vi "Node ID.vi"() -> ()   [LabVIEW 2016]
uses:
  Set Save Object Dictionary.vi
  Motor controllers.vi
  <vilib>/CANopenLib/CANOPEN.llb/CANopen SDO Create.vi
  Set node ID.vi
  Set PDOs COB IDs.vi
  Set COB EMCY ID.vi
  <vilib>/CANopenLib/CANOPEN.llb/CANopen SDO Write.vi
  <vilib>/CANopenLib/CANOPEN.llb/CANopen SDO Write [STR].vi
  <vilib>/CANopenLib/CANOPEN.llb/CANopen SDO Close.vi
  <vilib>/CANopenLib/CANOPEN.llb/CANopen Interface Close.vi
panel:
  in  "Motor":u8(ring) items=["Right", "Left"]
  in  "New Node ID":u8=1 min=1 max=127 step=1
  out "error out":errorcluster
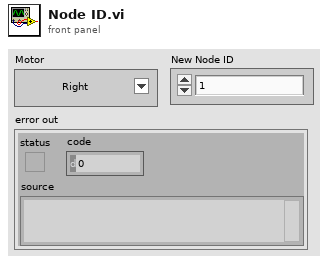
[diagram p1: front panel]
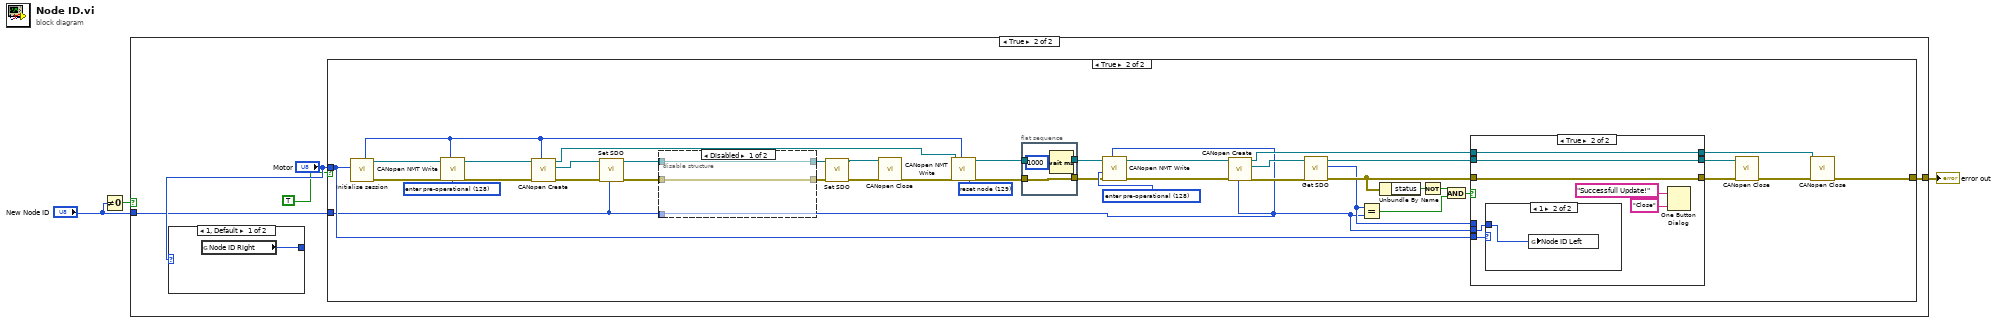
[diagram p0: block diagram]
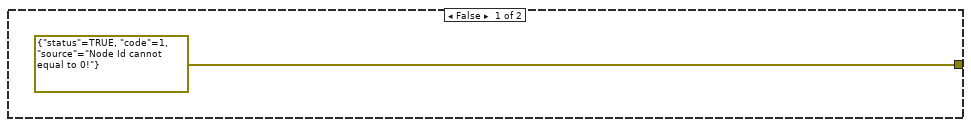
[diagram p2: hidden frame]
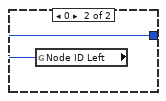
[diagram p3: hidden frame]
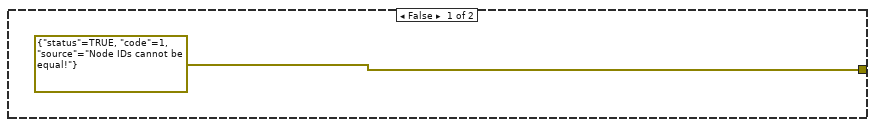
[diagram p4: hidden frame]
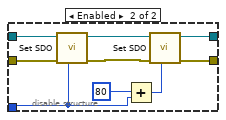
[diagram p5: hidden frame]
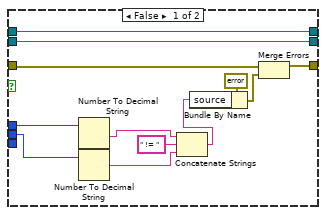
[diagram p6: hidden frame]
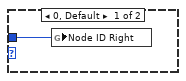
[diagram p7: hidden frame]
diagram:
  n1 = Not Equal To 0?(x="New Node ID") -> (x != 0?=w2:bool)
  n2 = case shown="True" w2 {
    tunnel: [errorcluster {"status"=TRUE, "code"=1, "source"="Node Id cannot equal to 0!"} ("error constant") w8] -> w3
    tunnel: "New Node ID" -> [_ w6]
    frame False {
    }
    frame True {
      n3 = case shown="1, Default" "Motor" {
        tunnel: [w9 w10] -> _
        frame 1, Default {
          n4 = global read "Motor controllers.vi" "Node ID Right"() -> (w9:u8)
        }
        frame 0 {
          n5 = global read "Motor controllers.vi" "Node ID Left"() -> (w10:u8)
        }
      }
      n6 = case shown="True" TRUE {
        tunnel: "Motor" -> [_ w49]
        tunnel: w6 -> [_ w16]
        tunnel: [errorcluster {"status"=TRUE, "code"=1, "source"="Node IDs cannot be equal!"} ("error constant") w35] -> w8
        frame False {
        }
        frame True {
          w21 = u16 128 items=["start remote node"=1, "stop remote node"=2, "enter pre-operational"=128, "reset node"=129, "reset communication"=130] ("command")
          w22 = u16 129 items=["start remote node"=1, "stop remote node"=2, "enter pre-operational"=128, "reset node"=129, "reset communication"=130] ("command")
          w50 = u16 128 items=["start remote node"=1, "stop remote node"=2, "enter pre-operational"=128, "reset node"=129, "reset communication"=130] ("command")
          n7 = call "Initialise session.vi"("Motor"=w49) -> ("error out"=w44:errorcluster, "interface object out"=w43:refnum<k20>, "Used Node ID"=w26:u8)  [unwired: 8 in]
          n8 = call <vilib>:"CANopen NMT Write.vi"("node-ID (0)"=w26, "error in (no error)"=w44, "command"=w50, "interface object in"=w43) -> ("error out"=w46:errorcluster, "interface object out"=w45:refnum<k20>)  [unwired: 6 in]
          n9 = call-poly <vilib>:"CANopen Create.vi"("node-ID"=w26, "error in (no error)"=w46, "interface object in"=w45) -> ("error out"=w52:errorcluster, "SDO object out"=w51:refnum<k20>, "interface object out"=w23:refnum<k20>)  [unwired: 6 in]
          n10 = call-poly "Set SDO.vi"("Node ID"=w16, "error in (no error)"=w52, "SDO object in"=w51) -> ("error out"=w20:errorcluster, "SDO object out"=w19:refnum<k20>)  [unwired: 6 in, 1 out]
          n11 = disable-structure shown="Disabled" {
            disable-tunnel: w20 -> [w53 w63]
            disable-tunnel: w19 -> [w54 w62]
            disable-tunnel: [w53 w59] -> w18
            disable-tunnel: [w54 w58] -> w17
            disable-tunnel: w16 -> [_ w56]
            frame Disabled {
            }
            frame Enabled {
              n12 = call-poly "Set SDO.vi"("Node ID"=w56, "error in (no error)"=w63, "SDO object in"=w62) -> ("error out"=w60:errorcluster, "SDO object out"=w61:refnum<k20>)  [unwired: 7 in]
              n13 = Add(x=u32 80, y=w56) -> (x+y=w55:u32)
              n14 = call-poly "Set SDO.vi"("COB EMCY ID"=w55, "error in (no error)"=w60, "SDO object in"=w61) -> ("error out"=w59:errorcluster, "SDO object out"=w58:refnum<k20>)  [unwired: 6 in, 1 out]
            }
          }
          n15 = call-poly "Set SDO.vi"("error in (no error)"=w18, "SDO object in"=w17) -> ("error out"=w28:errorcluster, "SDO object out"=w29:refnum<k20>)  [unwired: 7 in, 1 out]
          n16 = call-poly <vilib>:"CANopen Close.vi"("error in (no error)"=w28, "SDO object in"=w29) -> ("error out"=w27:errorcluster)  [unwired: 9 in]
          n17 = call <vilib>:"CANopen NMT Write.vi"("node-ID (0)"=w26, "error in (no error)"=w27, "command"=w22, "interface object in"=w23) -> ("error out"=w12:errorcluster, "interface object out"=w14:refnum<k20>)  [unwired: 6 in]
          n18 = flat-sequence {
            tunnel: [w66] -> w15
            tunnel: w14 -> [w66]
            tunnel: [w65] -> w13
            tunnel: w12 -> [w65]
            frame #0 {
              n19 = Wait (ms)(milliseconds to wait=u32 1000) -> ()  [unwired: 1 out]
            }
          }
          n20 = call <vilib>:"CANopen NMT Write.vi"("node-ID (0)"=w16, "error in (no error)"=w13, "command"=w21, "interface object in"=w15) -> ("error out"=w24:errorcluster, "interface object out"=w25:refnum<k20>)  [unwired: 6 in]
          n21 = call-poly <vilib>:"CANopen Create.vi"("node-ID"=w16, "error in (no error)"=w24, "interface object in"=w25) -> ("error out"=w47:errorcluster, "SDO object out"=w48:refnum<k20>, "interface object out"=w32:refnum<k20>)  [unwired: 6 in]
          n22 = call-poly "Get SDO.vi"("error in (no error)"=w47, "SDO object in"=w48) -> ("error out"=w38:errorcluster, "Node ID"=w30:u8, "SDO object out"=w39:refnum<k20>)  [unwired: 6 in, 1 out]
          n23 = Equal?(x=w30, y=w16) -> (x = y?=w41:bool)
          n24 = Unbundle By Name(w38) -> ("status"=w31:bool)
          n25 = Not(x=w31) -> (.not. x?=w42:bool)
          n26 = And(x=w42, y=w41) -> (x .and. y?=w40:bool)
          n27 = case shown="True" w40 {
            tunnel: [w78 w79] -> w37
            tunnel: w49 -> [_ w85]
            tunnel: w16 -> [w71 w84]
            tunnel: w39 -> [w77 w80]
            tunnel: w38 -> [w75 w79]
            tunnel: [w77 w80] -> w34
            tunnel: [w76 w81] -> w33
            tunnel: w32 -> [w76 w81]
            tunnel: w30 -> [w72 _]
            frame False {
              n28 = Number To Decimal String(number=w72) -> (decimal integer string=w69:string)  [unwired: 1 in]
              n29 = Number To Decimal String(number=w71) -> (decimal integer string=w68:string)  [unwired: 1 in]
              n30 = Concatenate Strings(w69, " != " ("string"), w68) -> (w67:string)
              n31 = Bundle By Name(cluster=errorcluster {"status"=TRUE, "code"=1, "source"=""} ("error constant"), "source"=w67) -> (w73:errorcluster)
              n32 = Merge Errors(w75, w73) -> (w78:errorcluster)
            }
            frame True {
              n33 = case shown="1" w85 {
                tunnel: w84 -> [w86 w87]
                frame 0, Default {
                  n34 = global write "Motor controllers.vi" "Node ID Right"(w86) -> ()
                }
                frame 1 {
                  n35 = global write "Motor controllers.vi" "Node ID Left"(w87) -> ()
                }
              }
              n36 = One Button Dialog(message="Successfull Update!", button name ("OK")="Close") -> ()  [unwired: 1 out]
            }
          }
          n37 = call-poly <vilib>:"CANopen Close.vi"("error in (no error)"=w37, "SDO object in"=w34) -> ("error out"=w36:errorcluster)  [unwired: 9 in]
          n38 = call-poly <vilib>:"CANopen Close.vi"("error in (no error)"=w36, "interface object in"=w33) -> ("error out"=w35:errorcluster)  [unwired: 9 in]
        }
      }
    }
  }
  "error out" <- w3
